vi "MotorInit.vi"(8 "error in (no error)":errorcluster) -> (0 "error out":errorcluster)   [LabVIEW 2015]
uses:
  <vilib>/Rock Robotics/WPI/CAN/TalonSRX/WPI_CANTalonSRX_APIFeedbackSelect.ctl
  <vilib>/Rock Robotics/WPI/CAN/TalonSRX/WPI_CANTalonSRX_APIControlMode.ctl
  Utilities/AutoVars.vi
  Utilities/VisionGlobals.vi
  Utilities/ShiftGlobals.vi
  Utilities/GlobalGyro.vi
  Utilities/GlobalVisionVars.vi
  Utilities/MotorPositionGlobals.vi
  Utilities/GeneralGlobals.vi
  navx-mxp/labview/navX Library v2/navX Library v2.lvlib
panel:
  in  "Manipulator PID Gains":T1={"proportional gain (Kc)"=3.0, "integral time (Ti, min)"=0.0, "derivative time (Td, min)"=5.0}
  in  "Drive PID Gains Position":T1={"proportional gain (Kc)"=3.0, "integral time (Ti, min)"=0.0, "derivative time (Td, min)"=7.0}
  in  "Drive PID Gains Velocity":T1={"proportional gain (Kc)"=0.5, "integral time (Ti, min)"=0.0, "derivative time (Td, min)"=1.0}
  in  "Tensioner PID Gains":T1={"proportional gain (Kc)"=3.0, "integral time (Ti, min)"=0.0, "derivative time (Td, min)"=4.0}
  in  "Winch PID Gains":T1={"proportional gain (Kc)"=10.0, "integral time (Ti, min)"=0.0, "derivative time (Td, min)"=4.0}
  in  "Arm PID Gains":T1={"proportional gain (Kc)"=2.0, "integral time (Ti, min)"=0.0, "derivative time (Td, min)"=6.0}
  # "10"
  # "4"
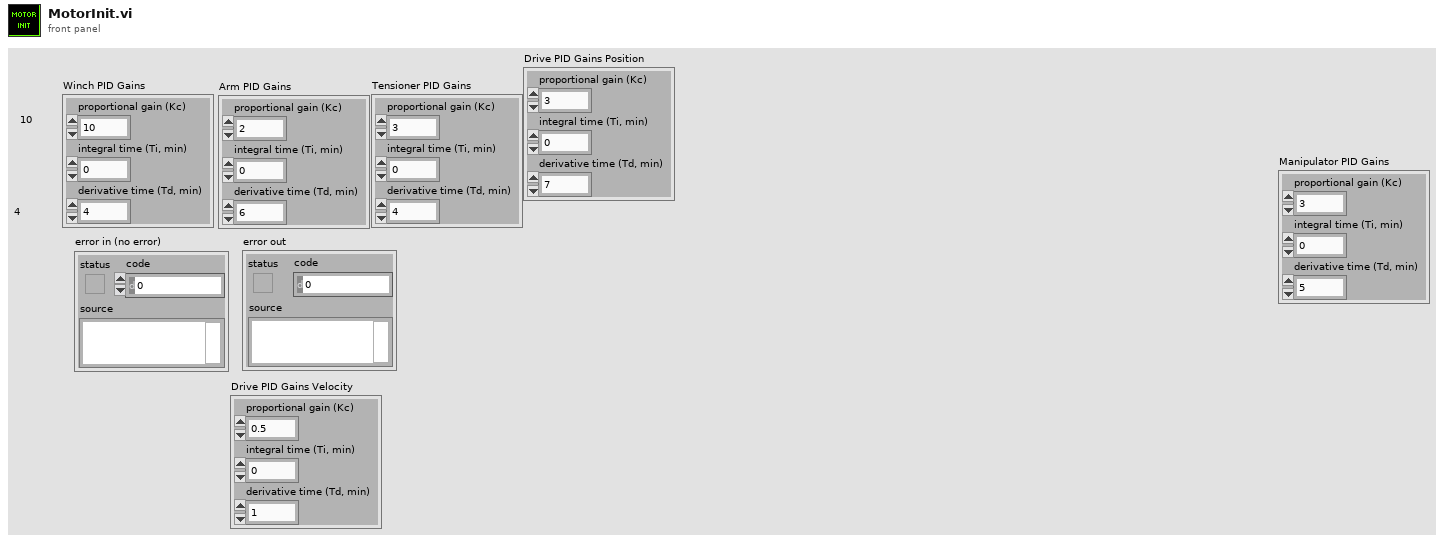
[diagram p1: front panel]
types:
  T1 = cluster{"proportional gain (Kc)":dbl, "integral time (Ti, min)":dbl, "derivative time (Td, min)":dbl}
  T2 = typedef "WPI_CANTalonSRX_APIControlMode.ctl" = enum8{"Percent VBus", "Speed", "Position", "Slave", "Unchanged / Invalid", "Voltage Compensation", "Current", "Motion Profile"}
  T3 = typedef "WPI_CANTalonSRX_APIFeedbackSelect.ctl" = enum16{"Digital Quadrature Encoder", "Analog Potentiometer", "Analog Encoder", "Count on Quad-A (Rising-Edge)", "Count on Quad-A (Falling-Edge)", "CTR Magnetic Enc (Absolute)", "CTR Magnetic Enc (Relative)", "Pulse Width"}
  T4 = typedef "navX Library v2.lvlib/Z900_navX_DeviceTypeDef.ctl" = cluster{"Interface":cluster{"Protocol":T5, "Update Rate (4Hz-100Hz)":u8, "navX Open TypeDef":variant}, "Notify Packet":refnum<notifier>, "Loop VI Refnum":refnum<vi>, "Ready to Close Occurrence Refnum":refnum<k4>}
  T5 = typedef "navX Library v2.lvlib/Z900_navX_ProtocolTypeDef.ctl" = enum16{"SERIAL", "I2C", "SPI"}
  T6 = typedef "WPI_MotorControlDeviceRef.ctl" = cluster{"DeviceStatus":errorcluster, "Type":T7, "PWM":cluster{"PWM Channel":T8, "DeadBand":T9}, "CAN":cluster{"Device Number":u8, "Control Mode":T10, "Semaphore":T11, "Max Vout":dbl, "TalonSRX Control Mode":T2}, "Invert":bool}
  T7 = typedef "WPI_MotorControlType.ctl" = enum16{"PWM", "CAN", "CANTalonSRX"}
  T8 = typedef "FPGA_DIOPWMChannel.ctl" = enum8{"PWM 0", "PWM 1", "PWM 2", "PWM 3", "PWM 4", "PWM 5", "PWM 6", "PWM 7", "PWM 8", "PWM 9", "PWM MXP 0", "PWM MXP 1", "PWM MXP 2", "PWM MXP 3", "PWM MXP 4", "PWM MXP 5", "PWM MXP 6", "PWM MXP 7", "PWM MXP 8", "PWM MXP 9", "Invalid"}
  T9 = typedef "WPI_PWMDeadband.ctl" = cluster{"Name":string, "maxPositivePwm":i32, "minPositivePwm":i32, "centerPwm":i32, "maxNegativePwm":i32, "minNegativePwm":i32, "angularRange":u16}
  T10 = typedef "WPI_CANJaguar_ControlMode.ctl" = enum8{"Percent VBus", "Current", "Speed", "Position", "Voltage"}
  T11 = typedef "Semaphore RefNum" = refnum<k1>
  T12 = typedef "WPI_SwitchDevRef.ctl" = cluster{"DevStatus":errorcluster, "DIO Channel":T13, "CntIndex":T14, "Normally Closed":bool}
  T13 = typedef "FPGA_DIOChannel.ctl" = enum8{"DIO 0", "DIO 1", "DIO 2", "DIO 3", "DIO 4", "DIO 5", "DIO 6", "DIO 7", "DIO 8", "DIO 9", "DIO MXP 0", "DIO MXP 1", "DIO MXP 2", "DIO MXP 3", "DIO MXP 4", "DIO MXP 5", "DIO MXP 6", "DIO MXP 7", "DIO MXP 8", "DIO MXP 9", "DIO MXP 10", "DIO MXP 11", "DIO MXP 12", "DIO MXP 13", "DIO MXP 14", "DIO MXP 15", "Invalid"}
  T14 = typedef "FPGA_CounterCtrSystemIndex.ctl" = enum8{"Ctr 0", "Ctr 1", "Ctr 2", "Ctr 3", "Ctr 4", "Ctr 5", "Ctr 6", "Ctr 7", "Invalid"}
  T15 = typedef "WPI_CANTalonSRX_GlobalStatus.ctl" = cluster{"Applied Throttle":dbl, "Module Enabled":bool, "CAN Error":errorcluster, "Closed Loop Error":dbl, "Forward Limit Switch Closed":bool, "Reverse Limit Switch Closed":bool, "Sensor Position":dbl, "Sensor Velocity":dbl, "Current":dbl, "Sticky Fault - Over Temp":bool, "Sticky Fault - Under Voltage":bool, "Sticky Fault - Forward Limit":bool, "Sticky Fault - Reverse Limit":bool, "Sticky Fault - Forward Soft Limit":bool, "Sticky Fault - Reverse Soft Limit":bool, "Brake is Enabled":bool, "Encoder Position":dbl, "Encoder Velocity":dbl, "Encoder Index Count":dbl, "Encoder A Pin State":bool, "Encoder B Pin State":bool, "Encoder Index Pin State":bool, "Analog In":dbl, "Analog In Velocity":dbl, "Temperature (C)":dbl, "Battery Voltage":dbl, "Control 5 Is Supported":bool, "Current Profile Slot Select":dbl, "Pos Div 8":bool, "Vel Div 4":bool, "Pulse Width Position":i32, "Pulse Width Velocity":i32, "Pulse Width Rise To Rise (us)":i32, "Pulse Width Rise To Fall (us)":i32, "Mot Prof Active Is Under Run":bool, "Mot Prof Active Has Under Run":bool, "Mot Prof Active Is Last":bool, "Mot Prof Active Velocity Only":bool, "Mot Prof Active Is Valid":bool, "Mot Prof Buffer Is Full":bool, "Mot Prof Active Profile Slot Select":i32, "Mot Prof NextID":i32, "Mot Prof Count":i32, "Mot Prof Active Velocity":dbl, "Mot Prof Active Position":dbl, "Mot Prof Output Enable":i32}
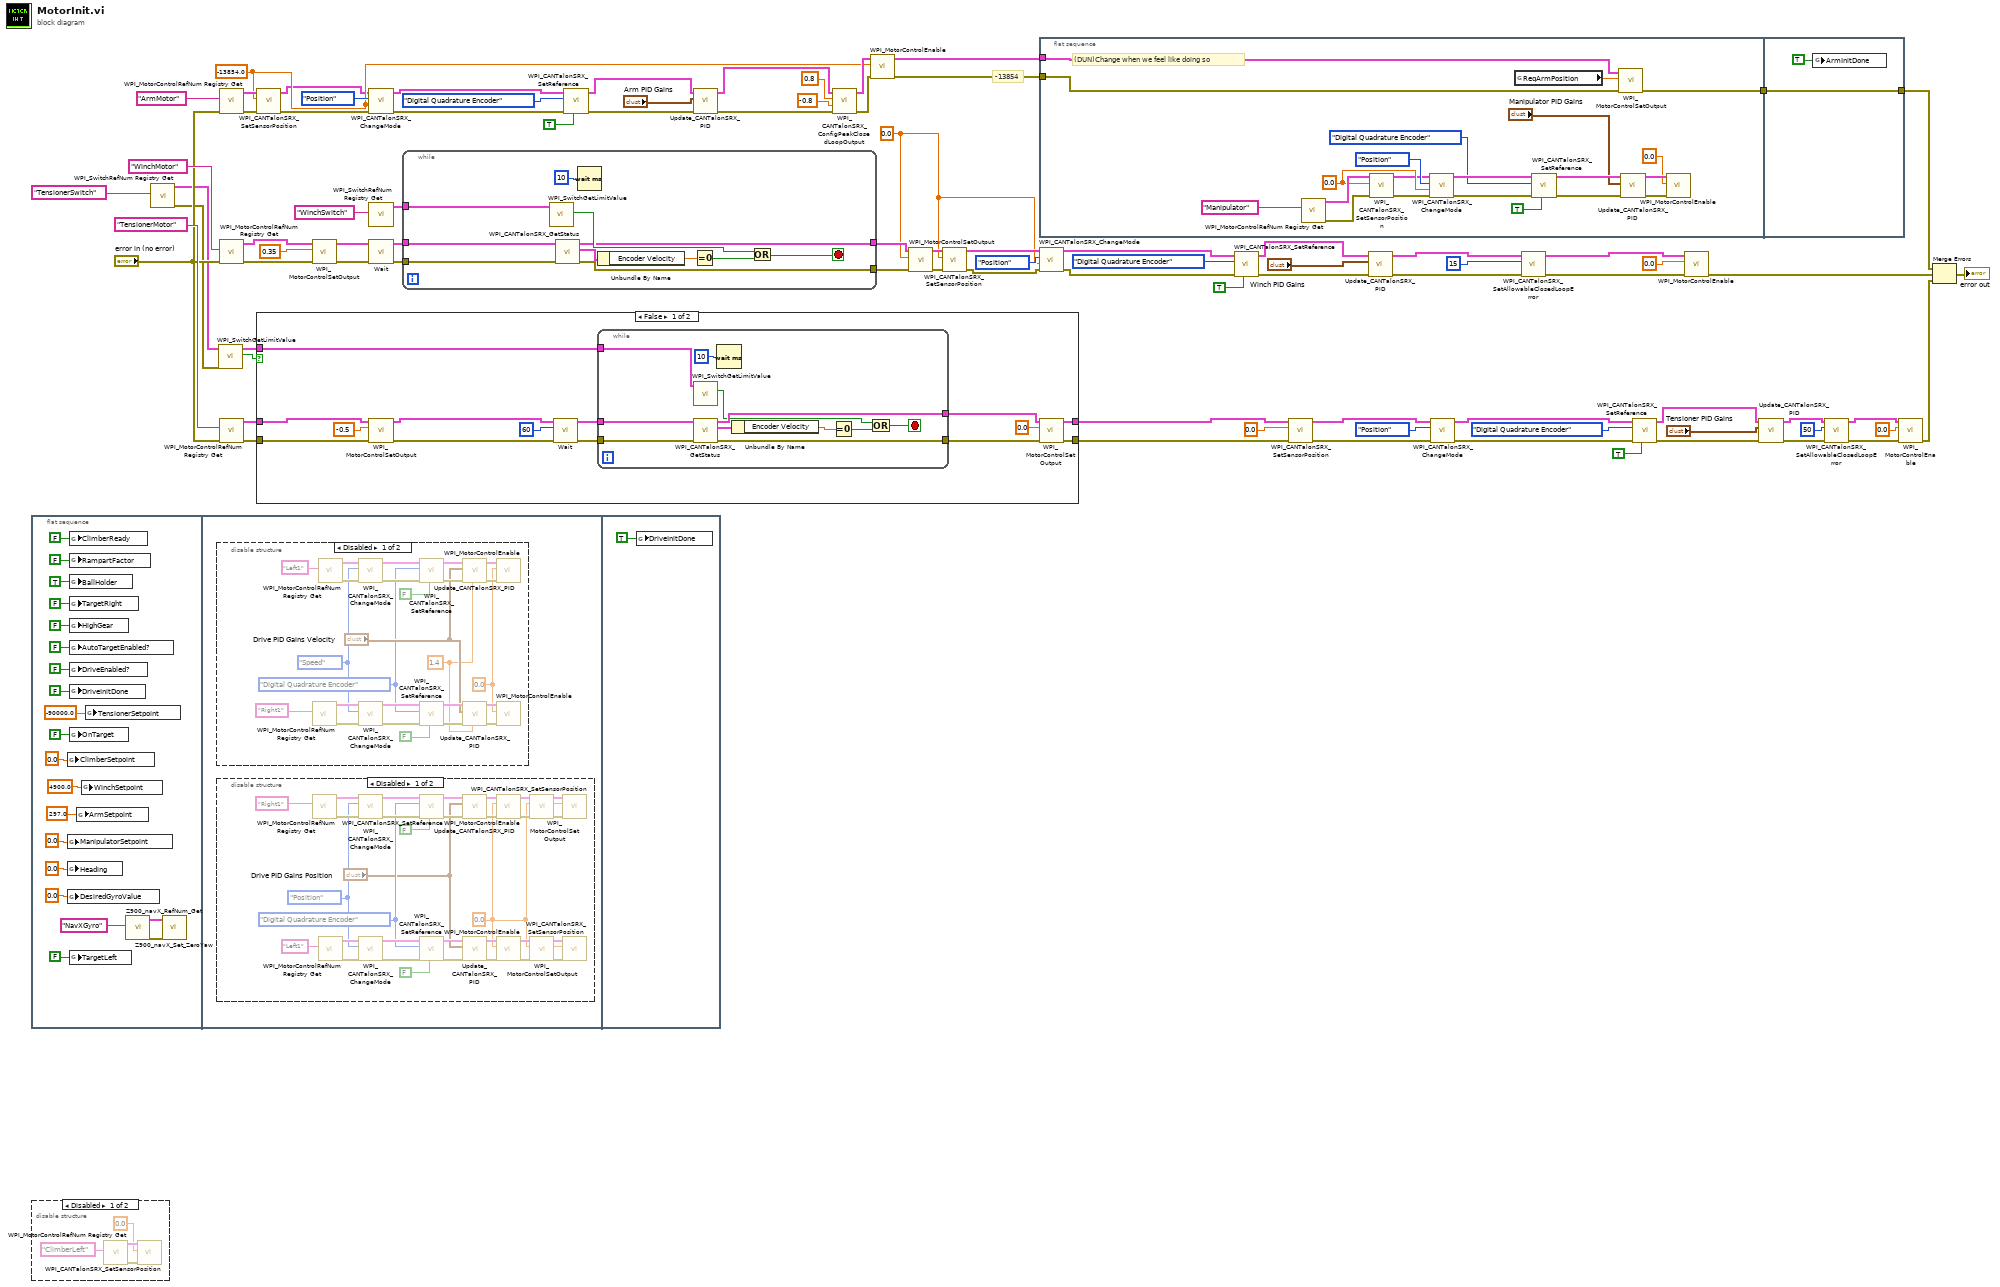
[diagram p0: block diagram]
diagram:
  w23 = -13854.0 ("Encoder Initial Position")
  w1 = 0.0 ("Output")
  # "-13854"
  n1 = flat-sequence {
    frame #0 {
      n2 = global write "MotorPositionGlobals.vi" "ClimberSetpoint"(0.0 ("ClimberSetpoint")) -> ()
      n3 = global write "MotorPositionGlobals.vi" "ManipulatorSetpoint"(0.0 ("ManipulatorSetpoint")) -> ()
      n4 = global write "GlobalVisionVars.vi" "Heading"(0.0 ("Heading")) -> ()
      n5 = global write "GlobalGyro.vi" "DesiredGyroValue"(0.0 ("DesiredGyroValue")) -> ()
      n6 = global write "GeneralGlobals.vi" "ClimberReady"(FALSE ("ClimberReady")) -> ()
      n7 = global write "AutoVars.vi" "RampartFactor"(FALSE ("RampartFactor")) -> ()
      n8 = global write "MotorPositionGlobals.vi" "BallHolder"(TRUE ("BallHolder")) -> ()
      n9 = global write "GlobalVisionVars.vi" "TargetRight"(FALSE ("OnTarget")) -> ()
      n10 = global write "ShiftGlobals.vi" "HighGear"(FALSE ("HighGear")) -> ()
      n11 = global write "VisionGlobals.vi" "AutoTargetEnabled?"(FALSE ("AutoTargetEnabled?")) -> ()
      n12 = global write "VisionGlobals.vi" "DriveEnabled?"(FALSE ("DriveEnabled?")) -> ()
      n13 = global write "AutoVars.vi" "DriveInitDone"(FALSE ("MotorInitDone")) -> ()
      n14 = global write "GlobalVisionVars.vi" "OnTarget"(FALSE ("OnTarget")) -> ()
      n15 = global write "GlobalVisionVars.vi" "TargetLeft"(FALSE ("OnTarget")) -> ()
      n16 = global write "MotorPositionGlobals.vi" "ArmSetpoint"(297.0 ("ArmSetpoint")) -> ()
      n17 = global write "MotorPositionGlobals.vi" "WinchSetpoint"(4900.0 ("WinchSetpoint")) -> ()
      n18 = global write "MotorPositionGlobals.vi" "TensionerSetpoint"(-90000.0 ("TensionerSetpoint")) -> ()
      n19 = call "Z900_navX_RefNum_Get.vi"("refnum name"="NavXGyro") -> ("error out"=w89:errorcluster, "navX Device"=w90:T4)  [unwired: 9 in]
      n20 = call "Z900_navX_Set_ZeroYaw.vi"("error in (no error)"=w89, "navX Device"=w90) -> ()  [unwired: 8 in, 2 out]
    }
    frame #1 {
      n21 = disable-structure shown="Disabled" {
        frame Disabled {
          w141 = 1.4 ("F")
          w146 = 0.0 ("Encoder Initial Position")
          w145 = WPI_CANTalonSRX_APIFeedbackSelect."Digital Quadrature Encoder" ("Feedback Reference")
          w144 = WPI_CANTalonSRX_APIControlMode."Speed" ("Control Mode")
          n22 = call <vilib>:"WPI_MotorControlRefNum Registry Get.vi"("refnum name"="Right1") -> ("error out"=w156:errorcluster, "MotorControlDevRef"=w157:T6)  [unwired: 9 in]
          n23 = call <vilib>:"WPI_MotorControlRefNum Registry Get.vi"("refnum name"="Left1") -> ("error out"=w148:errorcluster, "MotorControlDevRef"=w149:T6)  [unwired: 9 in]
          n24 = call <vilib>:"WPI_CANTalonSRX_ChangeMode.vi"("error in (no error)"=w148, "Control Mode"=w144, "CAN Talon SRX Ref"=w149) -> ("error out"=w154:errorcluster, "CAN Talon SRX Ref"=w155:T6)  [unwired: 7 in]
          n25 = call <vilib>:"WPI_CANTalonSRX_ChangeMode.vi"("error in (no error)"=w156, "Control Mode"=w144, "CAN Talon SRX Ref"=w157) -> ("error out"=w162:errorcluster, "CAN Talon SRX Ref"=w163:T6)  [unwired: 7 in]
          n26 = call <vilib>:"WPI_CANTalonSRX_SetReference.vi"("Reverse Closed-Loop Output"=FALSE, "error in (no error)"=w154, "Feedback Reference"=w145, "CAN Talon SRX Ref"=w155) -> ("error out"=w153:errorcluster, "CAN Talon SRX Ref"=w152:T6)  [unwired: 6 in]
          n27 = call <vilib>:"WPI_CANTalonSRX_SetReference.vi"("Reverse Closed-Loop Output"=FALSE, "error in (no error)"=w162, "Feedback Reference"=w145, "CAN Talon SRX Ref"=w163) -> ("error out"=w161:errorcluster, "CAN Talon SRX Ref"=w160:T6)  [unwired: 6 in]
          n28 = call "Update_CANTalonSRX_PID.vi"("F"=w141, "error in (no error)"=w153, "PID Gains"="Drive PID Gains Velocity", "CAN Talon SRX Ref"=w152) -> ("error out"=w151:errorcluster, "CAN Talon SRX Ref Out"=w150:T6)  [unwired: 6 in]
          n29 = call "Update_CANTalonSRX_PID.vi"("F"=w141, "error in (no error)"=w161, "PID Gains"="Drive PID Gains Velocity", "CAN Talon SRX Ref"=w160) -> ("error out"=w159:errorcluster, "CAN Talon SRX Ref Out"=w158:T6)  [unwired: 6 in]
          n30 = call <vilib>:"WPI_MotorControlEnable.vi"("error in (no error)"=w151, "Encoder Initial Position"=w146, "CAN MotorDevRef"=w150) -> ()  [unwired: 7 in, 2 out]
          n31 = call <vilib>:"WPI_MotorControlEnable.vi"("error in (no error)"=w159, "Encoder Initial Position"=w146, "CAN MotorDevRef"=w158) -> ()  [unwired: 7 in, 2 out]
        }
        frame Enabled {
        }
      }
      n32 = disable-structure shown="Disabled" {
        frame Disabled {
          w113 = 0.0 ("Encoder Initial Position")
          w122 = WPI_CANTalonSRX_APIFeedbackSelect."Digital Quadrature Encoder" ("Feedback Reference")
          w121 = WPI_CANTalonSRX_APIControlMode."Position" ("Control Mode")
          n33 = call <vilib>:"WPI_MotorControlRefNum Registry Get.vi"("refnum name"="Right1") -> ("error out"=w131:errorcluster, "MotorControlDevRef"=w132:T6)  [unwired: 9 in]
          n34 = call <vilib>:"WPI_MotorControlRefNum Registry Get.vi"("refnum name"="Left1") -> ("error out"=w123:errorcluster, "MotorControlDevRef"=w124:T6)  [unwired: 9 in]
          n35 = call <vilib>:"WPI_CANTalonSRX_ChangeMode.vi"("error in (no error)"=w131, "Control Mode"=w121, "CAN Talon SRX Ref"=w132) -> ("error out"=w137:errorcluster, "CAN Talon SRX Ref"=w138:T6)  [unwired: 7 in]
          n36 = call <vilib>:"WPI_CANTalonSRX_ChangeMode.vi"("error in (no error)"=w123, "Control Mode"=w121, "CAN Talon SRX Ref"=w124) -> ("error out"=w129:errorcluster, "CAN Talon SRX Ref"=w130:T6)  [unwired: 7 in]
          n37 = call <vilib>:"WPI_CANTalonSRX_SetReference.vi"("Reverse Closed-Loop Output"=FALSE, "error in (no error)"=w137, "Feedback Reference"=w122, "CAN Talon SRX Ref"=w138) -> ("error out"=w136:errorcluster, "CAN Talon SRX Ref"=w135:T6)  [unwired: 6 in]
          n38 = call <vilib>:"WPI_CANTalonSRX_SetReference.vi"("Reverse Closed-Loop Output"=FALSE, "error in (no error)"=w129, "Feedback Reference"=w122, "CAN Talon SRX Ref"=w130) -> ("error out"=w128:errorcluster, "CAN Talon SRX Ref"=w127:T6)  [unwired: 6 in]
          n39 = call "Update_CANTalonSRX_PID.vi"("error in (no error)"=w136, "PID Gains"="Drive PID Gains Position", "CAN Talon SRX Ref"=w135) -> ("error out"=w134:errorcluster, "CAN Talon SRX Ref Out"=w133:T6)  [unwired: 7 in]
          n40 = call "Update_CANTalonSRX_PID.vi"("error in (no error)"=w128, "PID Gains"="Drive PID Gains Position", "CAN Talon SRX Ref"=w127) -> ("error out"=w126:errorcluster, "CAN Talon SRX Ref Out"=w125:T6)  [unwired: 7 in]
          n41 = call <vilib>:"WPI_MotorControlEnable.vi"("error in (no error)"=w134, "Encoder Initial Position"=w113, "CAN MotorDevRef"=w133) -> ("error out"=w114:errorcluster, "CAN MotorDevRef"=w115:T6)  [unwired: 7 in]
          n42 = call <vilib>:"WPI_MotorControlEnable.vi"("error in (no error)"=w126, "Encoder Initial Position"=w113, "CAN MotorDevRef"=w125) -> ("error out"=w117:errorcluster, "CAN MotorDevRef"=w116:T6)  [unwired: 7 in]
          n43 = call <vilib>:"WPI_MotorControlSetOutput.vi"("error in (no error)"=w114, "Output"=w113, "MotorControlDevRef"=w115) -> ("error out"=w109:errorcluster, "Motor Output"=w108:dbl, "MotorControlDevRef"=w107:T6)  [unwired: 6 in]
          n44 = call <vilib>:"WPI_MotorControlSetOutput.vi"("error in (no error)"=w117, "Output"=w113, "MotorControlDevRef"=w116) -> ("error out"=w112:errorcluster, "Motor Output"=w111:dbl, "MotorControlDevRef"=w110:T6)  [unwired: 6 in]
          n45 = call <vilib>:"WPI_CANTalonSRX_SetSensorPosition.vi"("error in (no error)"=w109, "New Sensor Position"=w108, "CAN Talon SRX Ref"=w107) -> ()  [unwired: 7 in, 2 out]
          n46 = call <vilib>:"WPI_CANTalonSRX_SetSensorPosition.vi"("error in (no error)"=w112, "New Sensor Position"=w111, "CAN Talon SRX Ref"=w110) -> ()  [unwired: 7 in, 2 out]
        }
        frame Enabled {
        }
      }
    }
    frame #2 {
      n47 = global write "AutoVars.vi" "DriveInitDone"(TRUE ("MotorInitDone")) -> ()
    }
  }
  n48 = disable-structure shown="Disabled" {
    frame Disabled {
      n49 = call <vilib>:"WPI_MotorControlRefNum Registry Get.vi"("refnum name"="ClimberLeft") -> ("error out"=w169:errorcluster, "MotorControlDevRef"=w168:T6)  [unwired: 9 in]
      n50 = call <vilib>:"WPI_CANTalonSRX_SetSensorPosition.vi"("error in (no error)"=w169, "New Sensor Position"=0.0, "CAN Talon SRX Ref"=w168) -> ()  [unwired: 7 in, 2 out]
    }
    frame Enabled {
    }
  }
  n51 = call <vilib>:"WPI_SwitchRefNum Registry Get.vi"("refnum name"="TensionerSwitch") -> ("error out"=w33:errorcluster, "SwitchDevRef"=w36:T12)  [unwired: 9 in]
  n52 = call <vilib>:"WPI_SwitchGetLimitValue.vi"("error in (no error)"=w33, "SwitchDevRef"=w36) -> ("Switch Pressed"=w34:bool, "SwitchDevRef"=w35:T12)  [unwired: 7 in, 1 out]
  n53 = call <vilib>:"WPI_MotorControlRefNum Registry Get.vi"("error in (no error)"="error in (no error)", "refnum name"="ArmMotor") -> ("error out"=w25:errorcluster, "MotorControlDevRef"=w24:T6)  [unwired: 8 in]
  n54 = call <vilib>:"WPI_MotorControlRefNum Registry Get.vi"("error in (no error)"="error in (no error)", "refnum name"="WinchMotor") -> ("error out"=w83:errorcluster, "MotorControlDevRef"=w84:T6)  [unwired: 8 in]
  n55 = call <vilib>:"WPI_MotorControlRefNum Registry Get.vi"("error in (no error)"="error in (no error)", "refnum name"="TensionerMotor") -> ("error out"=w64:errorcluster, "MotorControlDevRef"=w63:T6)  [unwired: 8 in]
  n56 = call <vilib>:"WPI_CANTalonSRX_SetSensorPosition.vi"("error in (no error)"=w25, "New Sensor Position"=w23, "CAN Talon SRX Ref"=w24) -> ("error out"=w21:errorcluster, "CAN Talon SRX Ref"=w22:T6)  [unwired: 7 in]
  n57 = case shown="False" w34 {
    tunnel: w64 -> [w184 w196]
    tunnel: w63 -> [w183 w197]
    tunnel: [w179 w197] -> w15
    tunnel: [w178 w196] -> w16
    tunnel: w35 -> [w171 _]
    frame False {
      n58 = call <vilib>:"WPI_MotorControlSetOutput.vi"("error in (no error)"=w184, "Output"=-0.5, "MotorControlDevRef"=w183) -> ("error out"=w175:errorcluster, "MotorControlDevRef"=w176:T6)  [unwired: 6 in, 1 out]
      n59 = call "Wait.vi"("error in (no error)"=w175, "milliseconds to wait"=u32 60, "MotorControlDeviceRefIn"=w176) -> ("error out"=w173:errorcluster, "MotorControlDeviceRefOut"=w174:T6)  [unwired: 7 in]
      n60 = while {
        tunnel: w171 -> [w195]
        tunnel: [w189] -> w182
        tunnel: w174 -> [w191]
        tunnel: w173 -> [w190]
        tunnel: [w188] -> w181
        stop <- w186 stop-if-true
        n61 = call <vilib>:"WPI_SwitchGetLimitValue.vi"("SwitchDevRef"=w195) -> ("Switch Pressed"=w187:bool)  [unwired: 8 in, 2 out]
        n62 = call <vilib>:"WPI_CANTalonSRX_GetStatus.vi"("error in (no error)"=w190, "CAN Talon SRX Ref"=w191) -> ("error out"=w188:errorcluster, "Talon SRX Status"=w193:T15, "CAN Talon SRX Ref"=w189:T6)  [unwired: 7 in]
        n63 = Wait (ms)(milliseconds to wait=u32 10) -> ()  [unwired: 1 out]
        n64 = Unbundle By Name(w193) -> ("Encoder Velocity"=w192:dbl)
        n65 = Equal To 0?(x=w192) -> (x = 0?=w185:bool)
        n66 = Or(x=w187, y=w185) -> (x .or. y?=w186:bool)
      }
      n67 = call <vilib>:"WPI_MotorControlSetOutput.vi"("error in (no error)"=w181, "Output"=0.0, "MotorControlDevRef"=w182) -> ("error out"=w178:errorcluster, "MotorControlDevRef"=w179:T6)  [unwired: 6 in, 1 out]
    }
    frame True {
    }
  }
  n68 = call <vilib>:"WPI_MotorControlSetOutput.vi"("error in (no error)"=w83, "Output"=0.35, "MotorControlDevRef"=w84) -> ("error out"=w42:errorcluster, "MotorControlDevRef"=w43:T6)  [unwired: 6 in, 1 out]
  n69 = call <vilib>:"WPI_CANTalonSRX_ChangeMode.vi"("error in (no error)"=w21, "Output"=w23, "Control Mode"=WPI_CANTalonSRX_APIControlMode."Position", "CAN Talon SRX Ref"=w22) -> ("error out"=w53:errorcluster, "CAN Talon SRX Ref"=w54:T6)  [unwired: 6 in]
  n70 = call <vilib>:"WPI_SwitchRefNum Registry Get.vi"("refnum name"="WinchSwitch") -> ("SwitchDevRef"=w69:T12)  [unwired: 9 in, 1 out]
  n71 = call "Wait.vi"("error in (no error)"=w42, "MotorControlDeviceRefIn"=w43) -> ("error out"=w40:errorcluster, "MotorControlDeviceRefOut"=w41:T6)  [unwired: 8 in]
  n72 = while {
    tunnel: [w201] -> w79
    tunnel: [w200] -> w80
    tunnel: w69 -> [w208]
    tunnel: w41 -> [w199]
    tunnel: w40 -> [w198]
    stop <- w203 stop-if-true
    n73 = call <vilib>:"WPI_SwitchGetLimitValue.vi"("SwitchDevRef"=w208) -> ("Switch Pressed"=w207:bool)  [unwired: 8 in, 2 out]
    n74 = call <vilib>:"WPI_CANTalonSRX_GetStatus.vi"("error in (no error)"=w198, "CAN Talon SRX Ref"=w199) -> ("error out"=w200:errorcluster, "Talon SRX Status"=w206:T15, "CAN Talon SRX Ref"=w201:T6)  [unwired: 7 in]
    n75 = Wait (ms)(milliseconds to wait=u32 10) -> ()  [unwired: 1 out]
    n76 = Unbundle By Name(w206) -> ("Encoder Velocity"=w205:dbl)
    n77 = Equal To 0?(x=w205) -> (x = 0?=w202:bool)
    n78 = Or(x=w207, y=w202) -> (x .or. y?=w203:bool)
  }
  n79 = call <vilib>:"WPI_CANTalonSRX_SetReference.vi"("Reverse Closed-Loop Output"=TRUE, "error in (no error)"=w53, "Feedback Reference"=WPI_CANTalonSRX_APIFeedbackSelect."Digital Quadrature Encoder", "CAN Talon SRX Ref"=w54) -> ("error out"=w50:errorcluster, "CAN Talon SRX Ref"=w51:T6)  [unwired: 6 in]
  n80 = call "Update_CANTalonSRX_PID.vi"("error in (no error)"=w50, "PID Gains"="Arm PID Gains", "CAN Talon SRX Ref"=w51) -> ("error out"=w46:errorcluster, "CAN Talon SRX Ref Out"=w47:T6)  [unwired: 7 in]
  n81 = call <vilib>:"WPI_CANTalonSRX_ConfigPeakClosedLoopOutput.vi"("error in (no error)"=w46, "Reverse Peak Output"=-0.8, "Forward Peak Output"=0.8, "CAN Talon SRX Ref"=w47) -> ("error out"=w27:errorcluster, "CAN Talon SRX Ref"=w28:T6)  [unwired: 6 in]
  n82 = call <vilib>:"WPI_MotorControlEnable.vi"("error in (no error)"=w27, "Encoder Initial Position"=w23, "CAN MotorDevRef"=w28) -> ("error out"=w31:errorcluster, "CAN MotorDevRef"=w32:T6)  [unwired: 7 in]
  n83 = call <vilib>:"WPI_MotorControlSetOutput.vi"("error in (no error)"=w80, "Output"=w1, "MotorControlDevRef"=w79) -> ("error out"=w19:errorcluster, "MotorControlDevRef"=w20:T6)  [unwired: 6 in, 1 out]
  n84 = call <vilib>:"WPI_CANTalonSRX_SetSensorPosition.vi"("error in (no error)"=w19, "New Sensor Position"=w1, "CAN Talon SRX Ref"=w20) -> ("error out"=w17:errorcluster, "CAN Talon SRX Ref"=w18:T6)  [unwired: 7 in]
  n85 = flat-sequence {
    tunnel: [w227] -> w29
    tunnel: w32 -> [w229]
    tunnel: w31 -> [w228]
    tunnel: [w231] -> w30
    tunnel: w29 -> [w231]
    frame #0 {
      w211 = 0.0 ("Output")
      # "(DUN)Change when we feel like doing so"
      n86 = call <vilib>:"WPI_MotorControlRefNum Registry Get.vi"("refnum name"="Manipulator") -> ("error out"=w213:errorcluster, "MotorControlDevRef"=w212:T6)  [unwired: 9 in]
      n87 = call <vilib>:"WPI_CANTalonSRX_SetSensorPosition.vi"("error in (no error)"=w213, "New Sensor Position"=w211, "CAN Talon SRX Ref"=w212) -> ("error out"=w209:errorcluster, "CAN Talon SRX Ref"=w210:T6)  [unwired: 7 in]
      n88 = call <vilib>:"WPI_CANTalonSRX_ChangeMode.vi"("error in (no error)"=w209, "Output"=w211, "Control Mode"=WPI_CANTalonSRX_APIControlMode."Position", "CAN Talon SRX Ref"=w210) -> ("error out"=w222:errorcluster, "CAN Talon SRX Ref"=w223:T6)  [unwired: 6 in]
      n89 = global read "AutoVars.vi" "ReqArmPosition"() -> (w226:dbl)
      n90 = call <vilib>:"WPI_CANTalonSRX_SetReference.vi"("Reverse Closed-Loop Output"=TRUE, "error in (no error)"=w222, "Feedback Reference"=WPI_CANTalonSRX_APIFeedbackSelect."Digital Quadrature Encoder", "CAN Talon SRX Ref"=w223) -> ("error out"=w218:errorcluster, "CAN Talon SRX Ref"=w219:T6)  [unwired: 6 in]
      n91 = call <vilib>:"WPI_MotorControlSetOutput.vi"("error in (no error)"=w228, "Output"=w226, "MotorControlDevRef"=w229) -> ("error out"=w227:errorcluster)  [unwired: 6 in, 2 out]
      n92 = call "Update_CANTalonSRX_PID.vi"("error in (no error)"=w218, "PID Gains"="Manipulator PID Gains", "CAN Talon SRX Ref"=w219) -> ("error out"=w215:errorcluster, "CAN Talon SRX Ref Out"=w216:T6)  [unwired: 7 in]
      n93 = call <vilib>:"WPI_MotorControlEnable.vi"("error in (no error)"=w215, "Encoder Initial Position"=0.0, "CAN MotorDevRef"=w216) -> ()  [unwired: 7 in, 2 out]
    }
    frame #1 {
      n94 = global write "AutoVars.vi" "ArmInitDone"(TRUE ("ArmInitDone")) -> ()
    }
  }
  n95 = call <vilib>:"WPI_CANTalonSRX_ChangeMode.vi"("error in (no error)"=w17, "Output"=w1, "Control Mode"=WPI_CANTalonSRX_APIControlMode."Position", "CAN Talon SRX Ref"=w18) -> ("error out"=w76:errorcluster, "CAN Talon SRX Ref"=w77:T6)  [unwired: 6 in]
  n96 = call <vilib>:"WPI_CANTalonSRX_SetReference.vi"("Reverse Closed-Loop Output"=TRUE, "error in (no error)"=w76, "Feedback Reference"=WPI_CANTalonSRX_APIFeedbackSelect."Digital Quadrature Encoder", "CAN Talon SRX Ref"=w77) -> ("error out"=w74:errorcluster, "CAN Talon SRX Ref"=w73:T6)  [unwired: 6 in]
  n97 = call <vilib>:"WPI_CANTalonSRX_SetSensorPosition.vi"("error in (no error)"=w16, "New Sensor Position"=0.0, "CAN Talon SRX Ref"=w15) -> ("error out"=w12:errorcluster, "CAN Talon SRX Ref"=w13:T6)  [unwired: 7 in]
  n98 = call "Update_CANTalonSRX_PID.vi"("error in (no error)"=w74, "PID Gains"="Winch PID Gains", "CAN Talon SRX Ref"=w73) -> ("error out"=w11:errorcluster, "CAN Talon SRX Ref Out"=w10:T6)  [unwired: 7 in]
  n99 = call <vilib>:"WPI_CANTalonSRX_ChangeMode.vi"("error in (no error)"=w12, "Control Mode"=WPI_CANTalonSRX_APIControlMode."Position", "CAN Talon SRX Ref"=w13) -> ("error out"=w60:errorcluster, "CAN Talon SRX Ref"=w61:T6)  [unwired: 7 in]
  n100 = call <vilib>:"WPI_CANTalonSRX_SetAllowableClosedLoopError.vi"("error in (no error)"=w11, "Allowable Closed-Loop Error"=u16 15, "CAN Talon SRX Ref"=w10) -> ("error out"=w8:errorcluster, "CAN Talon SRX Ref"=w9:T6)  [unwired: 7 in]
  n101 = call <vilib>:"WPI_CANTalonSRX_SetReference.vi"("Reverse Closed-Loop Output"=TRUE, "error in (no error)"=w60, "Feedback Reference"=WPI_CANTalonSRX_APIFeedbackSelect."Digital Quadrature Encoder", "CAN Talon SRX Ref"=w61) -> ("error out"=w56:errorcluster, "CAN Talon SRX Ref"=w57:T6)  [unwired: 6 in]
  n102 = call <vilib>:"WPI_MotorControlEnable.vi"("error in (no error)"=w8, "Encoder Initial Position"=0.0, "CAN MotorDevRef"=w9) -> ("error out"=w66:errorcluster)  [unwired: 7 in, 1 out]
  n103 = call "Update_CANTalonSRX_PID.vi"("error in (no error)"=w56, "PID Gains"="Tensioner PID Gains", "CAN Talon SRX Ref"=w57) -> ("error out"=w6:errorcluster, "CAN Talon SRX Ref Out"=w5:T6)  [unwired: 7 in]
  n104 = call <vilib>:"WPI_CANTalonSRX_SetAllowableClosedLoopError.vi"("error in (no error)"=w6, "Allowable Closed-Loop Error"=u16 50, "CAN Talon SRX Ref"=w5) -> ("error out"=w3:errorcluster, "CAN Talon SRX Ref"=w4:T6)  [unwired: 7 in]
  n105 = call <vilib>:"WPI_MotorControlEnable.vi"("error in (no error)"=w3, "Encoder Initial Position"=0.0, "CAN MotorDevRef"=w4) -> ("error out"=w67:errorcluster)  [unwired: 7 in, 1 out]
  n106 = Merge Errors(w30, w66, w67) -> (→"error out":errorcluster)
